vi "Enable Synchronization Trigger Receiving.vi"(8 "error in (no error)":errorcluster, 11 "VISA resource name":refnum<visa-resource-name>) -> (0 "error out":errorcluster, 3 "VISA resource name out":refnum<visa-resource-name>)   [LabVIEW 2009, in "Agilent PSG MXG Series.lvlib"]
doc: "For signal generators designated as slaves in the multiple BBG synchronization setup, this control enables them to receive a one-time baseband synchronization event trigger from the master. The signal generator receives the trigger signal through the PAT TRIG connector.\n\nPrior to executing this function, ensure that the Dual ARB player of the master is off.\n\n<B>Notes:</B>\n(1) This VI is valid only in N5182A that installs <B>Option 651</B> or <B>Option 652</B> or <B>Option 654</B> (Internal baseband generator)."
uses:
  Agilent PSG MXG Series.lvlib
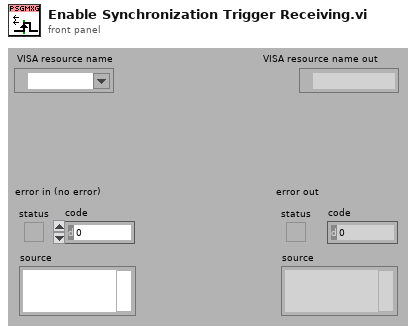
[diagram p1: front panel]
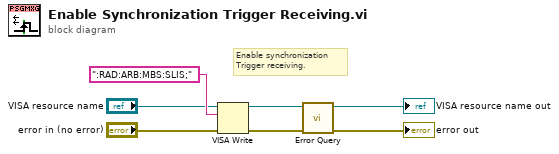
[diagram p0: block diagram]
diagram:
  # "Enable synchronization\nTrigger receiving."
  n1 = VISA Write(VISA resource name="VISA resource name", write buffer=":RAD:ARB:MBS:SLIS;", error in (no error)="error in (no error)") -> (VISA resource name out=w6:refnum<visa-resource-name>, error out=w5:errorcluster)  [unwired: 1 out]
  n2 = call "Error Query.vi"("error in (no error)"=w5, "VISA resource name"=w6) -> ("error out"=→"error out":errorcluster, "VISA resource name out"=→"VISA resource name out":refnum<visa-resource-name>)  [unwired: 8 out]
